vi "VI Test-Wet.vi"(6 "Zustand":T1=enum."ini", 8 "error in (no error)":errorcluster caption="Fehler (Eingang, kein Fehler)") -> (0 "error out":errorcluster caption="Fehler (Ausgang)", 3 "Status":string, 4 "Zustand":T1=enum."ini")   [LabVIEW 2020, in "EPA 1065.lvlib" / "Interference verificaton 1065-366.lvlib"]
uses:
  Interference verificaton 1065-366.lvlib
  Messdaten/Messdaten.lvlib
  Messdaten/Aktionen FGV Messdaten.ctl
  Aktion Test.ctl
  Seiten/FT-IR/FT-IR.lvlib
  Aktion FGV Interference.ctl
  Seiten/FT-IR/FGV FT-IR Aktionen.ctl
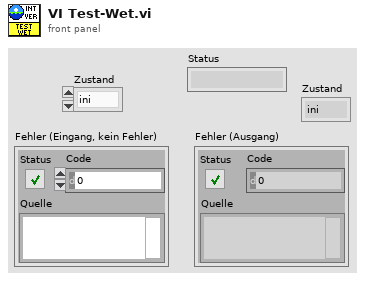
[diagram p1: front panel]
types:
  T1 = typedef "EPA 1065.lvlib/Interference verificaton 1065-366.lvlib/Aktion Test.ctl" = enum16{"Lesen", "ini", "ini - Konz", "Konzentration erreicht", "ini-warten", "Warten", "warten-aufzeichnen", "aufzeichnen", "ini-wet", "ini - konz - wet", "Konzentration erreicht - wet", "ini - warten - wet", "warten - wet", "warten - aufzeichnen - wet", "aufzeichnen - wet"}
  T2 = typedef "EPA 1065.lvlib/Interference verificaton 1065-366.lvlib/Aktion FGV Interference.ctl" = enum16{"Lesen", "Interference Daten", "Wert Dry schreiben", "Wert Wet schreiben", "VISA Schreiben"}
  T3 = typedef "FT-IR.lvlib/FGV FT-IR Aktionen.ctl" = enum16{"lesen", "NOG setzen", "NOS setzen", "Initialisieren", "speichern", "ALLES setzen", "FT-IR Spektrum loggen", "Komm Stoppen"}
  T4 = typedef "Messdaten.lvlib/Aktionen FGV Messdaten.ctl" = enum16{"lesen", "schreiben", "löschen", "Mittelwerte", "Komponente"}
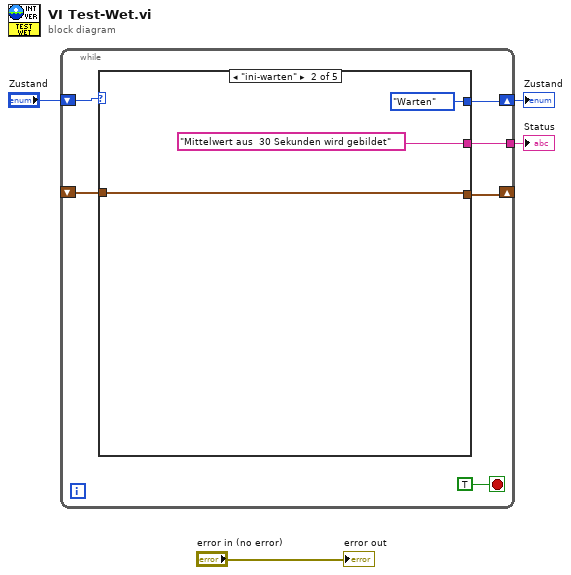
[diagram p0: block diagram]
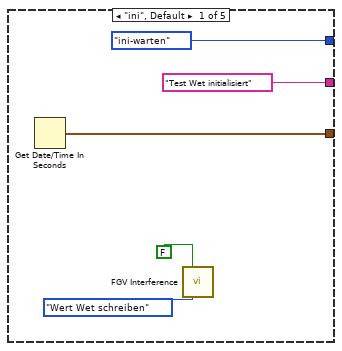
[diagram p2: hidden frame]
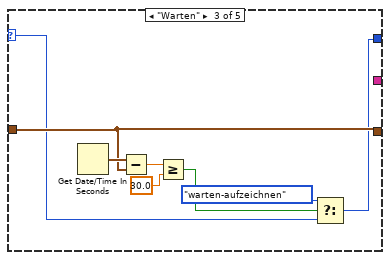
[diagram p3: hidden frame]
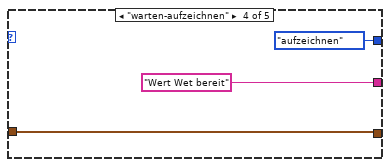
[diagram p4: hidden frame]
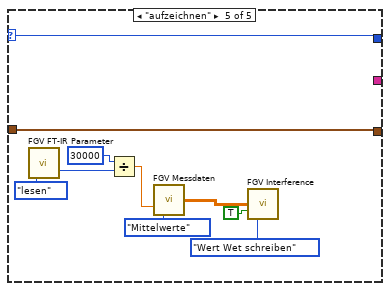
[diagram p5: hidden frame]
diagram:
  n1 = while {
    shift-right: [w9] -> _
    shift-left: _ -> [w8]
    shift-right: [w6] -> w3
    shift-left: "Zustand" -> [w7]
    tunnel: [w5] -> w1
    stop <- TRUE stop-if-true
    n2 = case shown="\"ini-warten\"" w7 {
      selector: w7 -> [_ _ w20 _ w34]
      tunnel: [w15 w16 w23 w27 w39] -> w9
      tunnel: w8 -> [_ w16 w23 w27 w39]
      tunnel: [Aktion_Test."ini-warten" ("Enum") Aktion_Test."Warten" ("Zustand") w19 Aktion_Test."aufzeichnen" ("Zustand") w34] -> w6
      tunnel: ["Test Wet initialisiert" "Mittelwert aus  30 Sekunden wird gebildet" _ "Wert Wet bereit" _] -> w5
      frame "ini", Default {
        n3 = Get Date/Time In Seconds() -> (seconds since 1Jan1904=w15:timestamp)
        n4 = call "FGV Interference.vi"(1:FALSE ("Boolesch"), "Aktion FGV Interference"=Aktion_FGV_Interference."Wert Wet schreiben") -> ()  [unwired: 10 in, 4 out]
      }
      frame "ini-warten" {
      }
      frame "Warten" {
        n5 = Get Date/Time In Seconds() -> (seconds since 1Jan1904=w25:timestamp)
        n6 = Subtract(x=w25, y=w23) -> (x-y=w26:dbl)
        n7 = Greater Or Equal?(x=w26, y=30.0) -> (x >= y?=w21:bool)
        n8 = Select(t=Aktion_Test."warten-aufzeichnen" ("Enum"), s=w21, f=w20) -> (s? t:f=w19:T1)
      }
      frame "warten-aufzeichnen" {
      }
      frame "aufzeichnen" {
        n9 = call "FGV FT-IR Parameter.vi"("Aktion"=FGV_FT-IR_Aktionen."lesen") -> ("Zykluszeit Messdatenverteiler"=w35:u32)  [unwired: 11 in, 7 out]
        n10 = Divide(x=30000, y=w35) -> (x/y=w36:dbl)
        n11 = call "FGV Messdaten.vi"("Mittelwerte"=w36, "Aktionen"=Aktionen_FGV_Messdaten."Mittelwerte") -> ("Mittelwertdaten"=w31:sgl[][])  [unwired: 5 in, 8 out]
        n12 = call "FGV Interference.vi"(7:w31, "Bereit Dry"=TRUE ("Boolesch"), "Aktion FGV Interference"=Aktion_FGV_Interference."Wert Wet schreiben") -> ()  [unwired: 9 in, 4 out]
      }
    }
  }
  "Zustand" <- w3
  "Status" <- w1
  "error out" <- "error in (no error)"
